vi "All Windows In.vi"(8 "error in (no error)":errorcluster, 11 "[MDI] Parent in":refnum<class "[MDI] Parent.lvclass">) -> (0 "error out":errorcluster, 3 "[MDI] Parent out":refnum<class "[MDI] Parent.lvclass">)   [LabVIEW 2020, in "[MDI] Parent.lvlib" / "[MDI] Parent.lvclass"]
uses:
  [MDI] Parent.lvclass
  [MDI] Parent.lvclass/[MDI] Parent.ctl
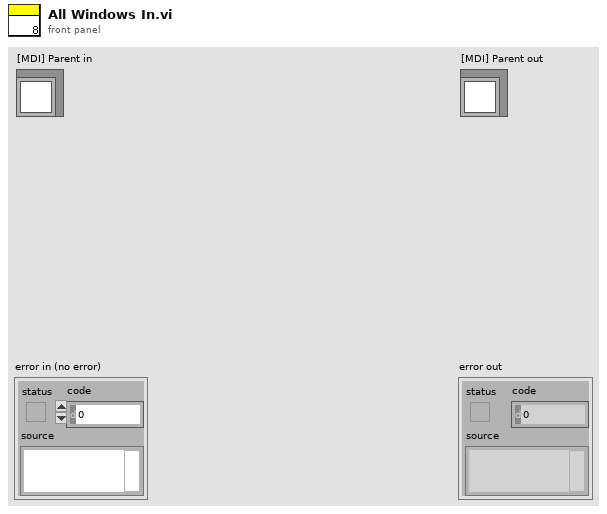
[diagram p1: front panel]
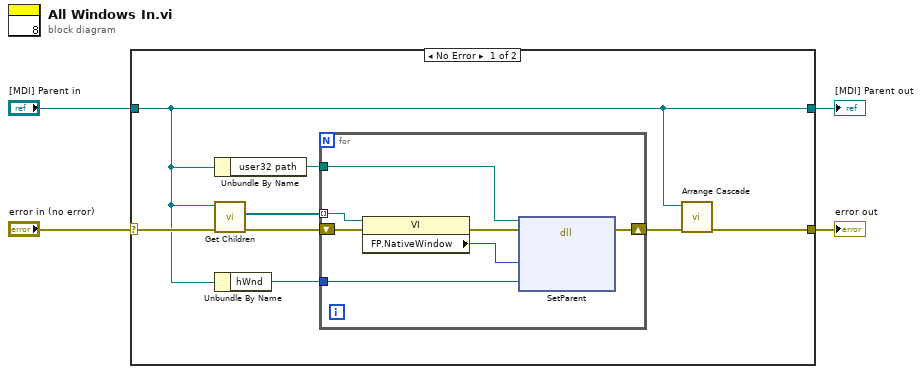
[diagram p0: block diagram]
diagram:
  n1 = case shown="No Error" "error in (no error)" {
    selector: "error in (no error)" -> [w12 w21]
    tunnel: [w7 w21] -> w3
    tunnel: [w6 w20] -> w1
    tunnel: "[MDI] Parent in" -> [w6 w20]
    frame No Error {
      n2 = Unbundle By Name(w6) -> ("user32 path"=w5:path)
      n3 = call "Get Children.vi"("error in (no error)"=w12, "[MDI] Parent in"=w6) -> ("error out"=w11:errorcluster, "all children"=w10:refnum<vi>[])  [unwired: 7 in, 1 out]
      n4 = Unbundle By Name(w6) -> ("hWnd"=w9:u32)
      n5 = for {
        shift-right: [w18] -> w8
        shift-left: w11 -> [w17]
        tunnel: w10 -> [w16] mode=indexing
        tunnel: w9 -> [w19]
        tunnel: w5 -> [w13]
        n6 = property class="VI"(reference=w16, error in=w17) -> (error out=w15:errorcluster, "FP.NativeWindow"=w14:u64)  [unwired: 1 out]
        n7 = dll-call lib="user32.dll" fn="SetParent"(path in=w13, error in=w15, "child"=w14, "newParent"=w19) -> (error out=w18:errorcluster)  [unwired: 4 in, 1 out]
      }
      n8 = call "Arrange Cascade.vi"("error in (no error)"=w8, "[MDI] Parent in"=w6) -> ("error out"=w7:errorcluster)  [unwired: 8 in, 1 out]
    }
    frame Error {
    }
  }
  "error out" <- w3
  "[MDI] Parent out" <- w1
